vi "SaveFile.vi"(10 "Name":string="Main.py", 11 "Code":string) -> (1 "file contents":string, 3 "Success?":bool)   [LabVIEW 2019]
panel:
  in  "Cancel Button":bool
  in  "OK Button":bool
  out "All strings":string[](array[string])
  # "Saving Code as:"
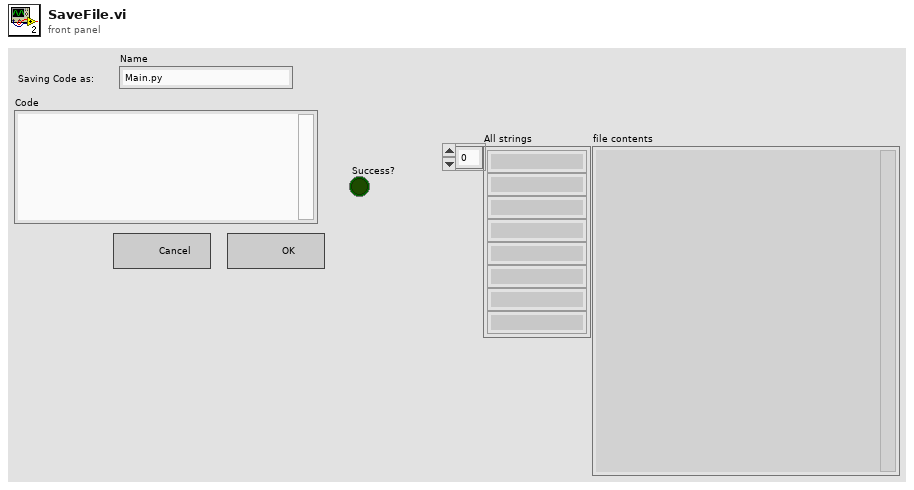
[diagram p1: front panel]
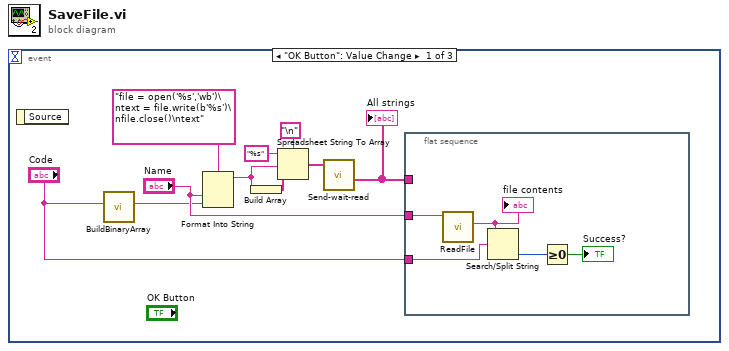
[diagram p0: block diagram]
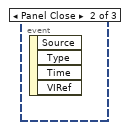
[diagram p2: hidden frame]
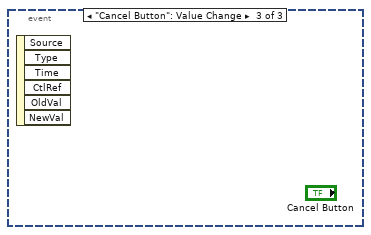
[diagram p3: hidden frame]
diagram:
  n1 = event shown="[0] \"OK Button\": Value Change" {
    selector: _ -> [_ _ _]
    dyn-events: _ -> [_ _ _]
    timeout: _ -> [_ _ _]
    event "OK Button": Value Change {
      n2 = event-data() -> ()  [unwired: 1 in, 1 out]
      n3 = call <userlib>:"BuildBinaryArray.vi"("String in"="Code") -> ("Binary String out"=w4:string)  [unwired: 10 in]
      n4 = Format Into String(format string="file = open('%s','wb')\ntext = file.write(b'%s')\nfile.close()\ntext" ("write buffer"), "Name", w4) -> (resulting string=w8:string)  [unwired: 2 in, 1 out]
      n5 = Build Array(w8) -> (w7:string[])
      n6 = Spreadsheet String To Array(delimiter (Tab)="\n", format string="%s", spreadsheet string=w8, array type (2D Dbl)=w7) -> (array=w9:string[])
      n7 = call "Send-wait-read.vi"("commands"=w9) -> ("All strings"=w2:string[])  [unwired: 9 in, 1 out]
      "All strings" <- w2
      n8 = flat-sequence {
        tunnel: "Code" -> [w15]
        tunnel: "Name" -> [w11]
        tunnel: w2 -> [_]
        frame #0 {
          n9 = call "ReadFile.vi"("String"=w11) -> ("file contents"=w14:string)  [unwired: 9 in, 1 out]
          "file contents" <- w14
          n10 = Search/Split String(string=w14, search string/char (-)=w15) -> (offset of match=w12:i32)  [unwired: 1 in, 2 out]
          n11 = Greater Or Equal To 0?(x=w12) -> (x >= 0?=→"Success?":bool)
        }
      }
    }
    event Panel Close {
      n12 = event-data() -> ()  [unwired: 1 in, 4 out]
    }
    event "Cancel Button": Value Change {
      n13 = event-data() -> ()  [unwired: 1 in, 6 out]
    }
  }
